vi "DAQ Hall Control.vi"(5 "Hall 5 Input":refnum<k21>, 6 "Hall 4 Input":refnum<k21>, 7 "Hall 3 Input":refnum<k21>, 8 "Hall 2 Input":refnum<k21>, 9 "Hall 1 Input":refnum<k21>, 10 "Control":u16) -> (0 "Hall 4 Output":refnum<k21>, 1 "Hall 5 Output":refnum<k21>, 2 "Hall 2 Output":refnum<k21>, 3 "Hall 1 Output":refnum<k21>, 4 "Hall 3 Output":refnum<k21>)   [LabVIEW 2023]
uses:
  <vilib>/DAQmx/write.llb/DAQmx Write (Digital Bool 1Line 1Point).vi
  <vilib>/DAQmx/miscellaneous.llb/DAQmx Fill In Error Info.vi
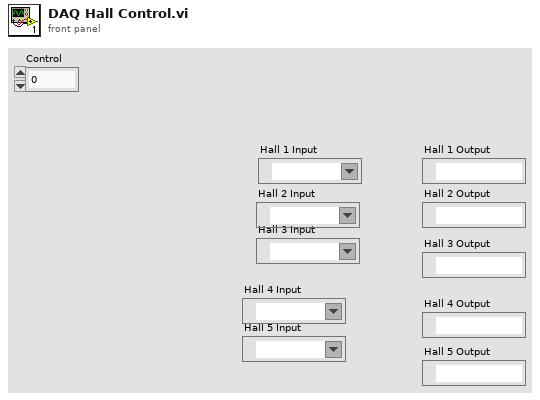
[diagram p1: front panel]
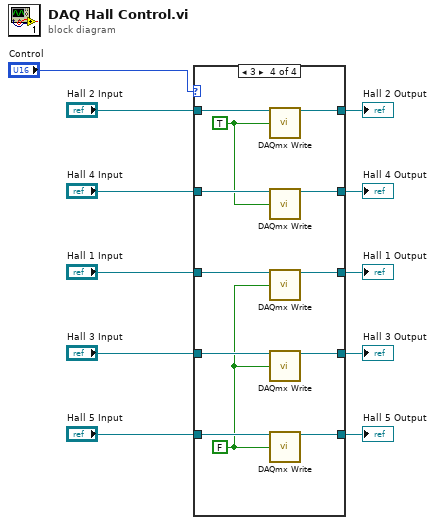
[diagram p0: block diagram]
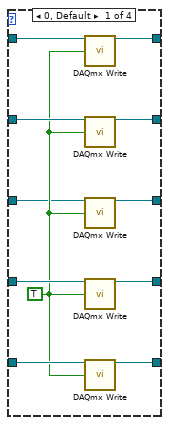
[diagram p2: hidden frame]
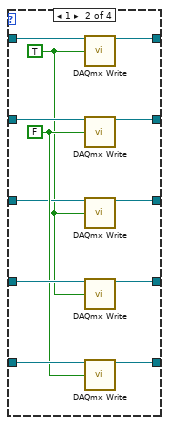
[diagram p3: hidden frame]
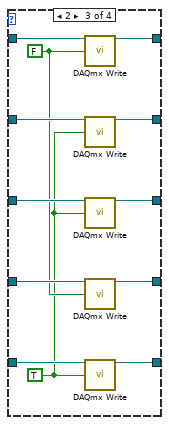
[diagram p4: hidden frame]
diagram:
  n1 = case shown="3" "Control" {
    tunnel: [w22 w34 w46 w58] -> w11
    tunnel: "Hall 5 Input" -> [w21 w33 w45 w57]
    tunnel: "Hall 4 Input" -> [w20 w32 w44 w56]
    tunnel: "Hall 3 Input" -> [w19 w31 w43 w55]
    tunnel: [w18 w30 w42 w54] -> w7
    tunnel: [w17 w29 w41 w53] -> w6
    tunnel: [w15 w27 w40 w52] -> w5
    tunnel: [w14 w26 w39 w51] -> w4
    tunnel: "Hall 2 Input" -> [w13 w25 w38 w50]
    tunnel: "Hall 1 Input" -> [w12 w24 w37 w49]
    frame 0, Default {
      w16 = TRUE ("data")
      n2 = call-poly <vilib>:"DAQmx Write.vi"("task/channels in"=w13, "data"=w16) -> ("task out"=w15:refnum<k21>)  [unwired: 11 in, 2 out]
      n3 = call-poly <vilib>:"DAQmx Write.vi"("task/channels in"=w20, "data"=w16) -> ("task out"=w18:refnum<k21>)  [unwired: 11 in, 2 out]
      n4 = call-poly <vilib>:"DAQmx Write.vi"("task/channels in"=w12, "data"=w16) -> ("task out"=w14:refnum<k21>)  [unwired: 11 in, 2 out]
      n5 = call-poly <vilib>:"DAQmx Write.vi"("task/channels in"=w19, "data"=w16) -> ("task out"=w17:refnum<k21>)  [unwired: 11 in, 2 out]
      n6 = call-poly <vilib>:"DAQmx Write.vi"("task/channels in"=w21, "data"=w16) -> ("task out"=w22:refnum<k21>)  [unwired: 11 in, 2 out]
    }
    frame 1 {
      w23 = TRUE
      w28 = FALSE ("data")
      n7 = call-poly <vilib>:"DAQmx Write.vi"("task/channels in"=w25, "data"=w23) -> ("task out"=w27:refnum<k21>)  [unwired: 11 in, 2 out]
      n8 = call-poly <vilib>:"DAQmx Write.vi"("task/channels in"=w32, "data"=w28) -> ("task out"=w30:refnum<k21>)  [unwired: 11 in, 2 out]
      n9 = call-poly <vilib>:"DAQmx Write.vi"("task/channels in"=w24, "data"=w23) -> ("task out"=w26:refnum<k21>)  [unwired: 11 in, 2 out]
      n10 = call-poly <vilib>:"DAQmx Write.vi"("task/channels in"=w31, "data"=w23) -> ("task out"=w29:refnum<k21>)  [unwired: 11 in, 2 out]
      n11 = call-poly <vilib>:"DAQmx Write.vi"("task/channels in"=w33, "data"=w28) -> ("task out"=w34:refnum<k21>)  [unwired: 11 in, 2 out]
    }
    frame 2 {
      w36 = FALSE
      w35 = TRUE ("data")
      n12 = call-poly <vilib>:"DAQmx Write.vi"("task/channels in"=w38, "data"=w36) -> ("task out"=w40:refnum<k21>)  [unwired: 11 in, 2 out]
      n13 = call-poly <vilib>:"DAQmx Write.vi"("task/channels in"=w44, "data"=w35) -> ("task out"=w42:refnum<k21>)  [unwired: 11 in, 2 out]
      n14 = call-poly <vilib>:"DAQmx Write.vi"("task/channels in"=w37, "data"=w35) -> ("task out"=w39:refnum<k21>)  [unwired: 11 in, 2 out]
      n15 = call-poly <vilib>:"DAQmx Write.vi"("task/channels in"=w43, "data"=w36) -> ("task out"=w41:refnum<k21>)  [unwired: 11 in, 2 out]
      n16 = call-poly <vilib>:"DAQmx Write.vi"("task/channels in"=w45, "data"=w35) -> ("task out"=w46:refnum<k21>)  [unwired: 11 in, 2 out]
    }
    frame 3 {
      w48 = FALSE
      w47 = TRUE ("data")
      n17 = call-poly <vilib>:"DAQmx Write.vi"("task/channels in"=w50, "data"=w47) -> ("task out"=w52:refnum<k21>)  [unwired: 11 in, 2 out]
      n18 = call-poly <vilib>:"DAQmx Write.vi"("task/channels in"=w56, "data"=w47) -> ("task out"=w54:refnum<k21>)  [unwired: 11 in, 2 out]
      n19 = call-poly <vilib>:"DAQmx Write.vi"("task/channels in"=w49, "data"=w48) -> ("task out"=w51:refnum<k21>)  [unwired: 11 in, 2 out]
      n20 = call-poly <vilib>:"DAQmx Write.vi"("task/channels in"=w55, "data"=w48) -> ("task out"=w53:refnum<k21>)  [unwired: 11 in, 2 out]
      n21 = call-poly <vilib>:"DAQmx Write.vi"("task/channels in"=w57, "data"=w48) -> ("task out"=w58:refnum<k21>)  [unwired: 11 in, 2 out]
    }
  }
  "Hall 5 Output" <- w11
  "Hall 4 Output" <- w7
  "Hall 3 Output" <- w6
  "Hall 2 Output" <- w5
  "Hall 1 Output" <- w4
